vi "SaveFileTest.vi"() -> ()   [LabVIEW 2023]
uses:
  <vilib>/numeric/sub_Random U32.vi
  <vilib>/express/express signal manip/GetorSetDDTAttributes/Set DDT Attributes/Set DDT Properties.xnode
  <vilib>/express/express shared/transition.llb/Dynamic To Waveform Array.vi
  <vilib>/express/express signal manip/GetorSetDDTAttributes/Set DDT Attributes/SetT0.vi
  <vilib>/express/express shared/transition.llb/Waveform Array To Dynamic.vi
panel:
  in  "Filename":path=path "test.xlsx"
  in  "Frequency":dbl
  in  "Power":dbl
  in  "Current":dbl
  in  "Voltage":dbl
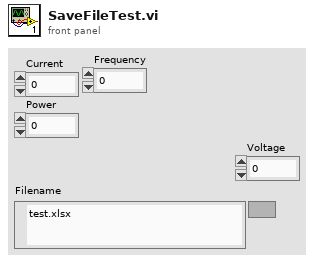
[diagram p1: front panel]
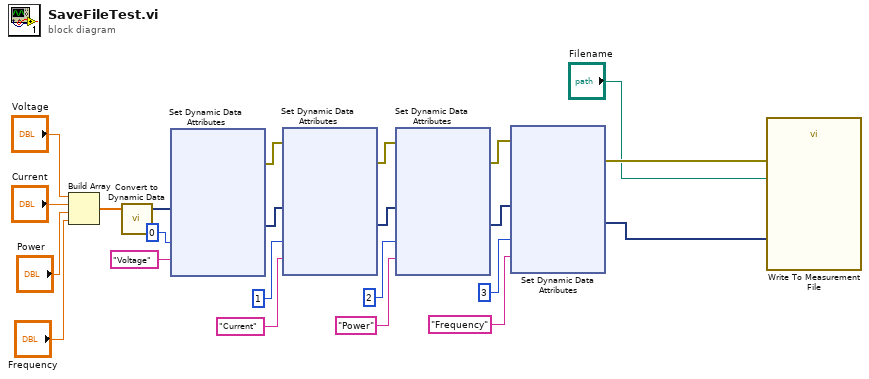
[diagram p0: block diagram]
diagram:
  n1 = Build Array("Voltage", "Current", "Power", "Frequency") -> (w19:dbl[])
  n2 = call "Convert to Dynamic Data"("Array"=w19) -> ("Dynamic Data Type"=w18:dynamicdata)  [unwired: 3 in]
  n3 = xnode "Set Dynamic Data Attributes"("Signals In"=w18, "Signal Index"=0, "Signal Name"="Voltage") -> ("Signals Out"=w13:dynamicdata, "error out"=w2:errorcluster)  [unwired: 1 in]
  n4 = xnode "Set Dynamic Data Attributes"("Signals In"=w13, "Signal Index"=1, "Signal Name"="Current", "error in"=w2) -> ("Signals Out"=w10:dynamicdata, "error out"=w3:errorcluster)
  n5 = xnode "Set Dynamic Data Attributes"("Signals In"=w10, "Signal Index"=2, "Signal Name"="Power", "error in"=w3) -> ("Signals Out"=w7:dynamicdata, "error out"=w4:errorcluster)
  n6 = xnode "Set Dynamic Data Attributes"("Signals In"=w7, "Signal Index"=3, "Signal Name"="Frequency", "error in"=w4) -> ("Signals Out"=w6:dynamicdata, "error out"=w5:errorcluster)
  n7 = call "Write To Measurement File"("Signals"=w6, "error in (no error)"=w5, "Filename"="Filename") -> ()  [unwired: 14 in, 3 out]
